vi "Get Test Members from Path.vi"(7 "application reference (local)":refnum<vi>, 8 "error in (no error)":errorcluster, 11 "Tests Path":path) -> (0 "error out":errorcluster, 2 "Test Members":path[](array[path]))   [LabVIEW 2009, in "GraphicalTestRunner.lvlib"]
uses:
  GraphicalTestRunner.lvlib
  <userlib>/_OpenG.lib/array/array.llb/Remove Duplicates from 1D Array (Path)__ogtk.vi
  <userlib>/_OpenG.lib/array/array.llb/Filter 1D Array with Scalar (Path)__ogtk.vi
  <userlib>/_OpenG.lib/array/array.llb/Conditional Auto-Indexing Tunnel (Path)__ogtk.vi
  <userlib>/_OpenG.lib/file/file.llb/Strip Path - Arrays__ogtk.vi
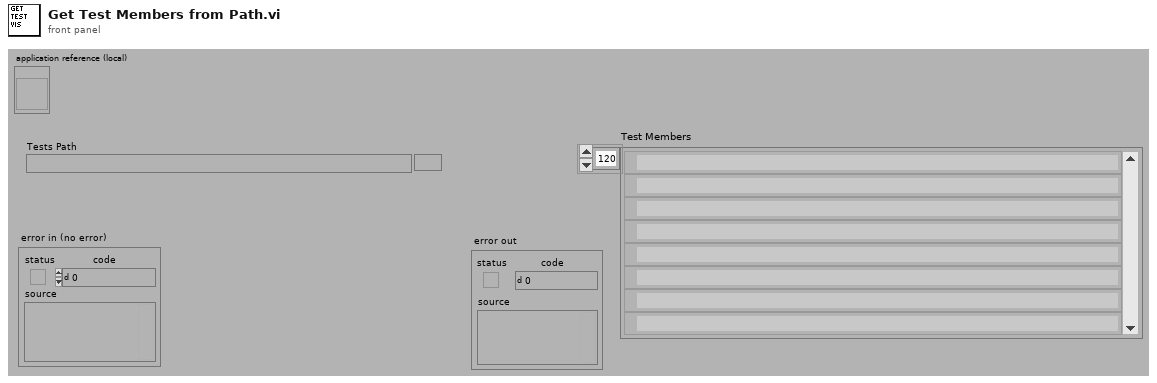
[diagram p1: front panel]
types:
  T1 = typedef "Liner Info - Cluster__jki_lib_application_control.ctl" = cluster{"path":path, "type":enum32{"Instrument", "Control", "CIN", "External subroutine", "Shared library", "Run-time menu", "Help file", "Palette menu"}, "iState":u32, "iStyle":u16, "wStyle":u16, "buttons":u16, "viflags":u32, "viflags2":u32, "links":u32[]}
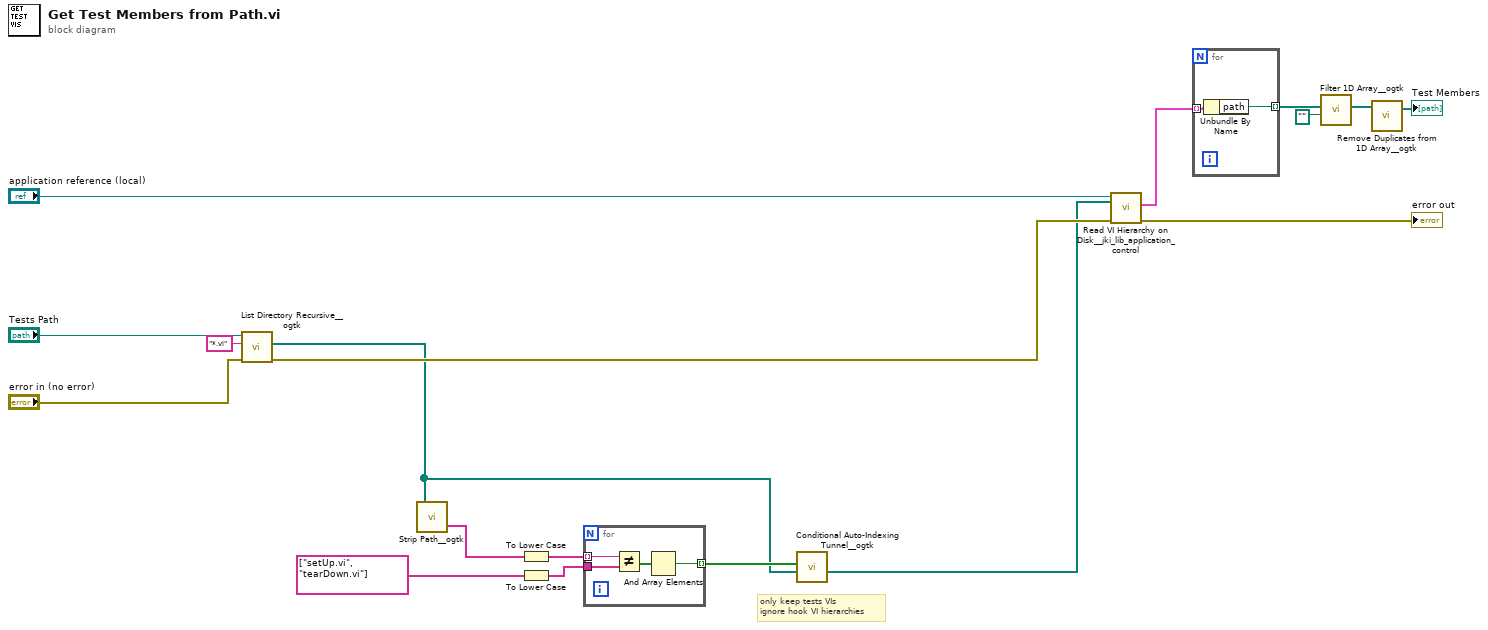
[diagram p0: block diagram]
diagram:
  # "only keep tests VIs\nignore hook VI hierarchies"
  n1 = call <userlib>:"List Directory Recursive__ogtk.vi"("error in (no error)"="error in (no error)", "pattern"="*.vi", "Path"="Tests Path") -> ("error out"=w12:errorcluster, "file paths"=w2:path[])  [unwired: 5 in, 2 out]
  n2 = call-poly <userlib>:"Strip Path__ogtk.vi"("path"=w2) -> ("name"=w7:string[])  [unwired: 1 out]
  n3 = To Lower Case(string=w7) -> (all lower case string=w6:string[])
  n4 = To Lower Case(string=string[] ["setUp.vi", "tearDown.vi"] ("y")) -> (all lower case string=w4:string[])
  n5 = for {
    tunnel: w6 -> [w22] mode=indexing
    tunnel: w4 -> [w21]
    tunnel: [w19] -> w3 mode=indexing
    n6 = Not Equal?(x=w22, y=w21) -> (x != y?=w20:bool[])
    n7 = And Array Elements(Boolean array=w20) -> (logical AND=w19:bool)
  }
  n8 = call-poly <userlib>:"Conditional Auto-Indexing Tunnel__ogtk.vi"("Array in"=w2, "Elements to keep"=w3) -> ("Filtered Array out"=w1:path[])  [unwired: 5 in]
  n9 = call <vilib>:"Read VI Hierarchy on Disk__jki_lib_application_control.vi"("error in"=w12, "Paths to Read"=w1, "application reference (local)"="application reference (local)") -> ("error out"=→"error out":errorcluster, "Linker Info"=w16:T1[])  [unwired: 5 in, 2 out]
  n10 = for {
    tunnel: w16 -> [w24] mode=indexing
    tunnel: [w23] -> w15 mode=indexing
    n11 = Unbundle By Name(w24) -> ("path"=w23:path)
  }
  n12 = call-poly <userlib>:"Filter 1D Array__ogtk.vi"("items to filter"=path "", "array"=w15) -> ("filtered array"=w17:path[])  [unwired: 4 in, 1 out]
  n13 = call-poly <userlib>:"Remove Duplicates from 1D Array__ogtk.vi"("Input Array"=w17) -> ("Output Array"=→"Test Members":path[])  [unwired: 1 out]
